vi "Draw Axes.vi"(11 "new picture in":picture) -> (3 "new picture out":picture)   [LabVIEW 2013]
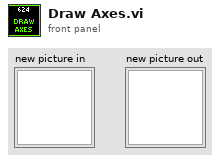
[diagram p1: front panel]
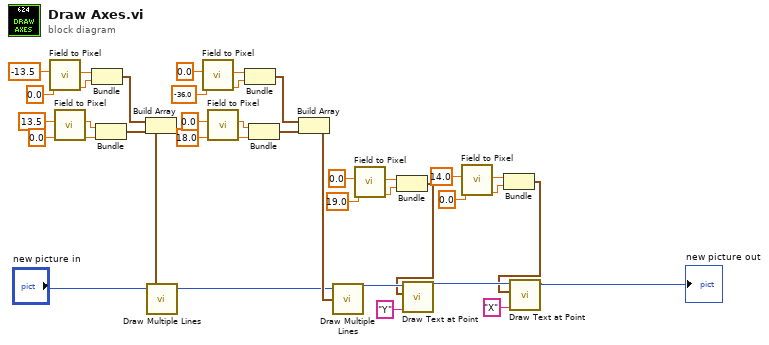
[diagram p0: block diagram]
diagram:
  n1 = call "Field to Pixel.vi"("Field Coordinate Y"=0.0, "Field Coordinate X"=-13.5) -> ("Pixel Y"=w18:dbl, "Pixel X"=w17:dbl)  [unwired: 8 in]
  n2 = call "Field to Pixel.vi"("Field Coordinate Y"=0.0, "Field Coordinate X"=13.5) -> ("Pixel Y"=w20:dbl, "Pixel X"=w21:dbl)  [unwired: 8 in]
  n3 = Bundle("Pixel X"=w17, "Pixel Y"=w18) -> (w19:cluster{"Pixel X":dbl, "Pixel Y":dbl})  [unwired: 1 in]
  n4 = Bundle("Pixel X"=w21, "Pixel Y"=w20) -> (w22:cluster{"Pixel X":dbl, "Pixel Y":dbl})  [unwired: 1 in]
  n5 = Build Array(w19, w22) -> (w16:cluster{"Pixel X":dbl, "Pixel Y":dbl}[])
  n6 = call <vilib>:"Draw Multiple Lines.vi"("picture"="new picture in", "line endpoints"=w16) -> ("new picture"=w38:picture)  [unwired: 7 in]
  n7 = call "Field to Pixel.vi"("Field Coordinate Y"=-36.0, "Field Coordinate X"=0.0) -> ("Pixel Y"=w36:dbl, "Pixel X"=w37:dbl)  [unwired: 8 in]
  n8 = call "Field to Pixel.vi"("Field Coordinate Y"=18.0, "Field Coordinate X"=0.0) -> ("Pixel Y"=w34:dbl, "Pixel X"=w33:dbl)  [unwired: 8 in]
  n9 = Bundle("Pixel X"=w37, "Pixel Y"=w36) -> (w35:cluster{"Pixel X":dbl, "Pixel Y":dbl})  [unwired: 1 in]
  n10 = Bundle("Pixel X"=w33, "Pixel Y"=w34) -> (w32:cluster{"Pixel X":dbl, "Pixel Y":dbl})  [unwired: 1 in]
  n11 = Build Array(w35, w32) -> (w39:cluster{"Pixel X":dbl, "Pixel Y":dbl}[])
  n12 = call <vilib>:"Draw Multiple Lines.vi"("picture"=w38, "line endpoints"=w39) -> ("new picture"=w15:picture)  [unwired: 7 in]
  n13 = call "Field to Pixel.vi"("Field Coordinate Y"=19.0, "Field Coordinate X"=0.0) -> ("Pixel Y"=w11:dbl, "Pixel X"=w10:dbl)  [unwired: 8 in]
  n14 = Bundle("Pixel X"=w10, "Pixel Y"=w11) -> (w9:cluster{"Pixel X":dbl, "Pixel Y":dbl})  [unwired: 1 in]
  n15 = call <vilib>:"Draw Text at Point.vi"("text"="Y", "origin"=w9, "picture"=w15) -> ("new picture"=w4:picture)  [unwired: 7 in, 1 out]
  n16 = call "Field to Pixel.vi"("Field Coordinate Y"=0.0, "Field Coordinate X"=14.0) -> ("Pixel Y"=w7:dbl, "Pixel X"=w8:dbl)  [unwired: 8 in]
  n17 = Bundle("Pixel X"=w8, "Pixel Y"=w7) -> (w2:cluster{"Pixel X":dbl, "Pixel Y":dbl})  [unwired: 1 in]
  n18 = call <vilib>:"Draw Text at Point.vi"("text"="X", "origin"=w2, "picture"=w4) -> ("new picture"=→"new picture out":picture)  [unwired: 7 in, 1 out]
